vi "Configure Session.vi"(8 "error in":errorcluster, 11 "Plugin in":refnum<class "Sequencer with Output Values.lvclass">) -> (0 "error out":errorcluster, 3 "Plugin out":refnum<class "Sequencer with Output Values.lvclass">)   [LabVIEW 2024, in "Sequencer with Output Values.lvlib" / "Sequencer with Output Values.lvclass"]
uses:
  Sequencer with Output Values.lvclass
  C:/Program Files/National Instruments/LabVIEW 2024/vi.lib/FlexLogger/SDK/PluginSDK.lvlibp/PEFClasses/SDK/Plugin/Plugin.lvclass
  Sequencer with Output Values.lvclass/Sequencer with Output Values.ctl
  <vilib>/FlexLogger/SDK/PluginSDK.lvlibp/PEFClasses/SDK/Producer Channel/Producer Channel.lvclass
  C:/Program Files/National Instruments/LabVIEW 2024/vi.lib/FlexLogger/SDK/PluginSDK.lvlibp/PEFClasses/SDK/Channel/Channel.lvclass
  Global Strings.vi
  <vilib>/FlexLogger/SDK/PluginSDK.lvlibp/PEFClasses/SDK/Plugin/ParameterAccess/Read String.vi
  <vilib>/FlexLogger/SDK/PluginSDK.lvlibp/PEFClasses/SDK/Plugin/Plugin.lvclass
  <vilib>/FlexLogger/SDK/PluginSDK.lvlibp
  C:/Program Files/National Instruments/LabVIEW 2024/vi.lib/FlexLogger/SDK/PluginSDK.lvlibp/PEFClasses/SDK/Processing Element/Processing Element.lvclass
  C:/dev/niflexlogger-plugins/plugins/Sequencer with Output Values/source/Sequencer with Output Values/Sequencer with Output Values.lvclass
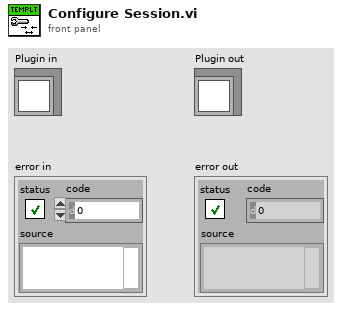
[diagram p1: front panel]
types:
  T1 = typedef "Sequencer with Output Values.lvlib/Sequencer with Output Values.lvclass/Params.ctl" = cluster{"Step Values":T2[], "Only Execute When Test Running":bool, "Reset Sequence When Test Starts":bool, "Current Sequence ID":u32, "Total Iterations":u32, "Last Timestamp":dbl, "Number of Sequence Steps":i32, "Num of Analog Channels":i32, "Num of Digital Channels":i32, "Delay Before Starting Sequence":dbl, "Changed":bool}
  T2 = typedef "Sequencer with Output Values.lvlib/Sequencer with Output Values.lvclass/Step Settings.ctl" = cluster{"Duration":dbl, "Mode":string, "Delay Between Values":dbl, "Analog Values":string[], "Digital Values":string[]}
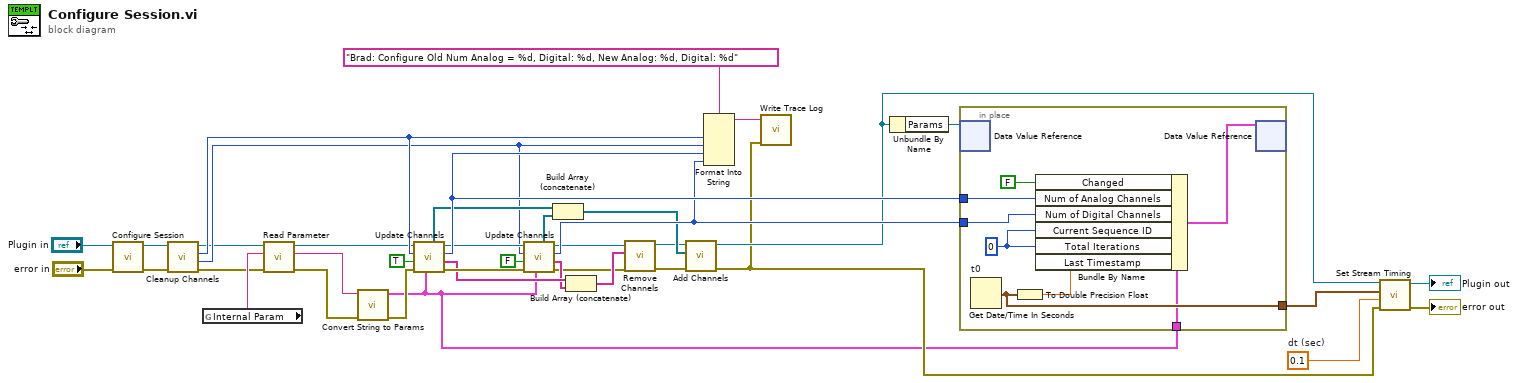
[diagram p0: block diagram]
diagram:
  w36 = 0.1  # dt (sec)
  n1 = call-parent "Configure Session.vi"("error in (no error)"="error in", "Processing Element in"="Plugin in") -> ("error out"=w6:errorcluster, "Processing Element out"=w22:refnum<class "Sequencer with Output Values.lvclass">)  [unwired: 8 in]
  n2 = call "Cleanup Channels.vi"("error in (no error)"=w6, "Plugin In"=w22) -> ("error out"=w2:errorcluster, "Num of Digital Channels"=w4:i32, "Num of Analog Channels"=w5:i32, "Plugin out"=w3:refnum<class "Sequencer with Output Values.lvclass">)  [unwired: 6 in]
  n3 = global read "Global Strings.vi" "Internal Param"() -> (w25:string)
  n4 = call-poly <vilib>:"Read Parameter.vi"("error in (no error)"=w2, "Name"=w25, "Plugin in"=w3) -> ("error out"=w7:errorcluster, "Value"=w23:string, "Plugin out"=w1:refnum<class "Sequencer with Output Values.lvclass">)  [unwired: 5 in, 1 out]
  n5 = call "Convert String to Params.vi"("error in (no error)"=w7, "String In"=w23) -> ("error out"=w24:errorcluster, "Param Out"=w8:T1)  [unwired: 8 in]
  n6 = call "Update Channels.vi"("Settings"=w8, "error in"=w24, "Analog"=TRUE, "Previous Number of Channels"=w5, "Plugin in"=w1) -> ("error out"=w27:errorcluster, "Channels to Remove"=w17:string[], "Updated Number of Channels"=w32:i32, "Plugin out"=w28:refnum<class "Sequencer with Output Values.lvclass">, "Channels to Add"=w20:refnum<class "Producer Channel.lvclass">[])  [unwired: 2 in]
  n7 = call "Update Channels.vi"("Settings"=w8, "error in"=w27, "Analog"=FALSE, "Previous Number of Channels"=w4, "Plugin in"=w28) -> ("error out"=w13:errorcluster, "Channels to Remove"=w16:string[], "Updated Number of Channels"=w31:i32, "Plugin out"=w14:refnum<class "Sequencer with Output Values.lvclass">, "Channels to Add"=w19:refnum<class "Producer Channel.lvclass">[])  [unwired: 2 in]
  n8 = Build Array (concatenate)(w20, w19) -> (w18:refnum<class "Producer Channel.lvclass">[])
  n9 = Build Array (concatenate)(w17, w16) -> (w15:string[])
  n10 = call-dynamic "Remove Channels.vi"("error in (no error)"=w13, "Unique Channel Identifiers to Delete"=w15, "Plugin in"=w14) -> ("error out"=w11:errorcluster, "Plugin out"=w12:refnum<class "Sequencer with Output Values.lvclass">)  [unwired: 7 in]
  n11 = call <vilib>:"Add Channels.vi"("error in (no error)"=w11, "Channels"=w18, "Plugin in"=w12) -> ("error out"=w9:errorcluster, "Plugin out"=w10:refnum<class "Sequencer with Output Values.lvclass">)  [unwired: 7 in]
  n12 = Format Into String(format string="Brad: Configure Old Num Analog = %d, Digital: %d, New Analog: %d, Digital: %d", w5, w4, w32, w31) -> (resulting string=w30:string)  [unwired: 2 in, 1 out]
  n13 = call <vilib>:"Write Trace Log.vi"("error in (no error)"=w9, "Message"=w30) -> ()  [unwired: 9 in, 1 out]
  n14 = Unbundle By Name(w10) -> ("Params"=w35:refnum<data-value>)
  n15 = in-place {
    in-place-border: [w45] -> w34
    in-place-border: w32 -> [w41]
    in-place-border: w31 -> [w43]
    in-place-border: w8 -> [w40]
    w46 = u32 0 ("Current Sequence ID")
    n16 = in-place-dvr #1(w35) -> ()  [unwired: 2 out]
    n17 = Get Date/Time In Seconds "t0"() -> (seconds since 1Jan1904=w45:timestamp)
    n18 = To Double Precision Float(number=w45) -> (double precision float=w44:dbl)
    n19 = Bundle By Name(cluster=w40, "Changed"=FALSE, "Num of Analog Channels"=w41, "Num of Digital Channels"=w43, "Current Sequence ID"=w46, "Total Iterations"=w46, "Last Timestamp"=w44) -> (w47:T1)
    n20 = in-place-dvr #1(w47) -> ()  [unwired: 2 out]
  }
  n21 = call-dynamic "Set Stream Timing.vi"("error in (no error)"=w9, "dt(sec)"=w36, "Start Time"=w34, "Plugin in"=w10) -> ("error out"=→"error out":errorcluster, "Plugin out"=→"Plugin out":refnum<class "Sequencer with Output Values.lvclass">)  [unwired: 6 in]
